vi "ATSpectrograph_logEvent_fwState.vi"(8 "error in (no error)":errorcluster, 11 "logevent_fwState_Ctl":T1) -> (0 "error out":errorcluster, 2 "function return":i32, 3 "logevent_fwState_Ctl out":T1)   [LabVIEW 2016, in "SALLV_ATSpectrograph.lvlib"]
doc: "int ATSpectrograph_shm_logEvent_fwStateLV(ATSpectrograph_logevent_fwStateLV *logevent_fwState_Ctl );"
uses:
  SALLV_ATSpectrograph.lvlib
  DataTypes/logevent_fwState.ctl
  SALLV_ATSpectrograph.so
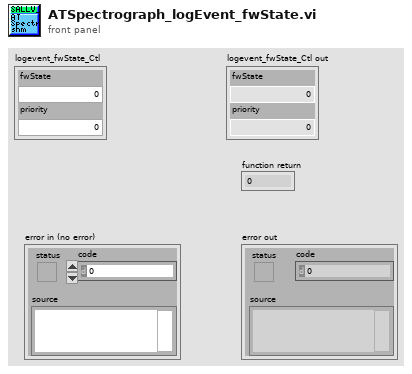
[diagram p1: front panel]
types:
  T1 = typedef "SALLV_ATSpectrograph.lvlib/logevent_fwState.ctl" = cluster{"fwState":i32, "priority":i32}
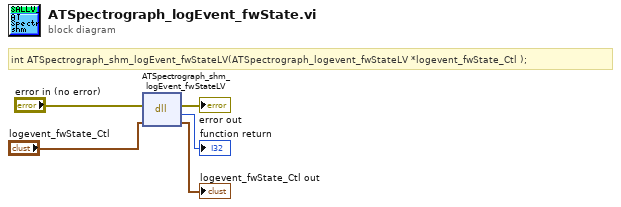
[diagram p0: block diagram]
diagram:
  # "int ATSpectrograph_shm_logEvent_fwStateLV(ATSpectrograph_logevent_fwStateLV *logevent_fwState_Ctl );"
  n1 = dll-call lib="home/harini/tcs/SALLV_ATSpectrograph/SALLV_ATSpectrograph.*" fn="ATSpectrograph_shm_logEvent_fwStateLV"(error in="error in (no error)", "logevent_fwState_Ctl"="logevent_fwState_Ctl") -> (error out=→"error out":errorcluster, →"function return":i32, "logevent_fwState_Ctl"=→"logevent_fwState_Ctl out":T1)  [unwired: 2 in, 1 out]
